vi "2D-Array search.vi"(7 "Cluster":T1, 9 "2D-String-Array_in":string[][](array[string])=[["45245,25", "Hallo", "Eier"], ["45245,36", "Ballo", "Mehl"], ["45245,84", "Lallo", "Zucker"], ["245", "Trallo", "Salz"], ["45", "Knallo", "Bier"]]) -> (1 "2D-String-Array_gefiltert":string[][](array[string]))   [LabVIEW 2020, in "allgemeine Sub-VIs.lvlib"]
uses:
  allgemeine Sub-VIs.lvlib
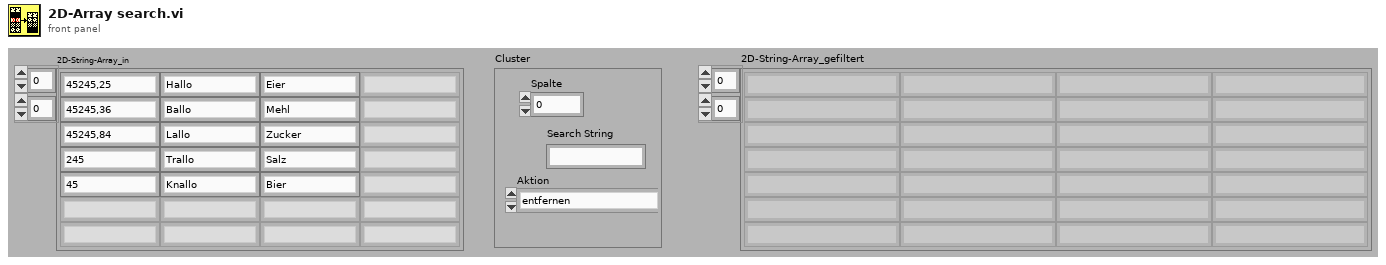
[diagram p1: front panel]
types:
  T1 = cluster{"Spalte":i32, "Search String":string, "Aktion":enum16{"entfernen", "nur diese belassen"}}
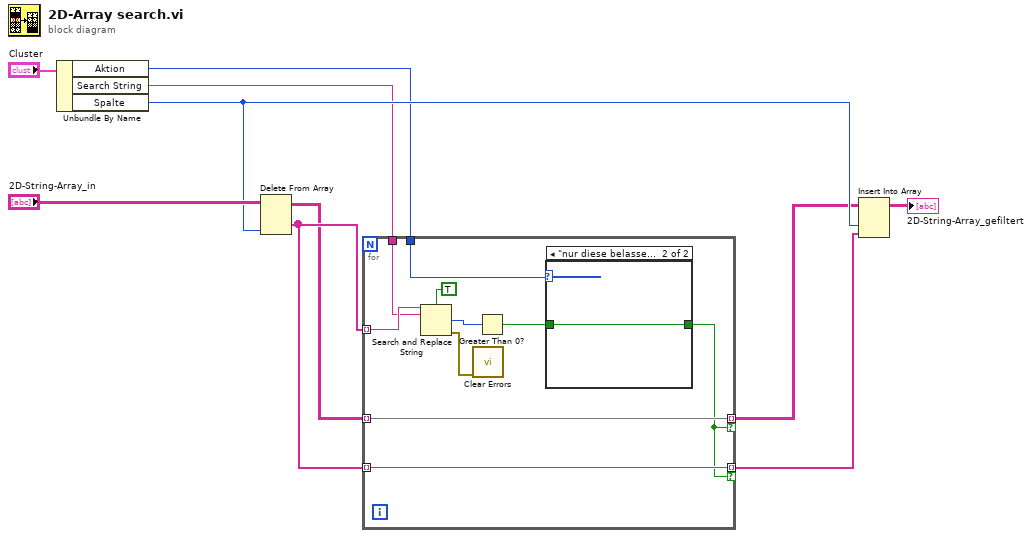
[diagram p0: block diagram]
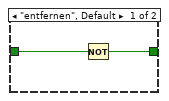
[diagram p2: hidden frame]
diagram:
  n1 = Unbundle By Name("Cluster") -> ("Aktion"=w6:enum16{"entfernen", "nur diese belassen"}, "Search String"=w7:string, "Spalte"=w8:i32)
  n2 = Delete From Array(array="2D-String-Array_in", index (col)=w8) -> (deleted portion=w5:string[], array with subset deleted=w4:string[][])  [unwired: 2 in]
  n3 = for {
    tunnel: w5 -> [w15] mode=indexing
    tunnel: w7 -> [w14]
    tunnel: w6 -> [w20]
    tunnel: w5 -> [w17] mode=indexing
    tunnel: [w17] -> w2 mode=indexing if=w16
    tunnel: w4 -> [w18] mode=indexing
    tunnel: [w18] -> w3 mode=indexing if=w16
    n4 = Search and Replace String(case sensitive?=TRUE ("Schreibweise ignorieren (F)"), input string=w15, search string=w14) -> (number of replacements=w13:i32, error out=w12:errorcluster)  [unwired: 5 in, 2 out]
    n5 = call <vilib>:"Clear Errors.vi"("error in (no error)"=w12) -> ()  [unwired: 5 in, 2 out]
    n6 = Greater Than 0?(x=w13) -> (x > 0?=w19:bool)
    n7 = case shown="\"nur diese belassen\"" w20 {
      tunnel: w19 -> [w22 w23]
      tunnel: [w21 w23] -> w16
      frame "entfernen", Default {
        n8 = Not(x=w22) -> (.not. x?=w21:bool)
      }
      frame "nur diese belassen" {
      }
    }
  }
  n9 = Insert Into Array(array=w3, index (col)=w8, new element=w2) -> (→"2D-String-Array_gefiltert":string[][])  [unwired: 1 in]
